vi "Main FPGA.vi"() -> ()   [LabVIEW 2019]
uses:
  Program Files (x86)/National Instruments/LabVIEW 2019/examples/CompactRIO/FPGA Fundamentals/FPGA Math and Analysis/FFT/Type Definitions/Windows.ctl
  <vilib>/Platform/TimedLoop/XDataNode/timing_clust.ctl
  <vilib>/Platform/TimedLoop/XDataNode/nitl_modes.ctl
  <vilib>/Platform/TimedLoop/XDataNode/wakeup.ctl
  <vilib>/rvi/Analysis/measure/FFT/simModelSupport/niFPGA FFT Sim Properties.ctl
  <vilib>/rvi/Analysis/measure/FFT/simModelSupport/niFPGA FFT Sim Types.ctl
  <vilib>/rvi/Analysis/measure/FFT/simModelSupport/niFpgaFFTSimArithmeticProperties.ctl
  <vilib>/rvi/Analysis/measure/FFT/simModelSupport/niFpgaFFTSimDfxp.ctl
  <vilib>/fxp/LVFixedPointQuantizationPolicyTypeDef.ctl
  <vilib>/rvi/Emulation/niFpgaGetClockAttributes.vi
  <vilib>/rvi/Emulation/niFpgaSctlEmulationGetInTimedLoop.vi
  <vilib>/rvi/Emulation/niFpgaEmulationReportErrorSimple.vi
  <vilib>/rvi/Emulation/niFpgaProcessEmulError.vi
  <vilib>/rvi/eio/common/nirviEmuTemplateMethod_errors.vi
  <vilib>/rvi/DataTransferAndStorage/Container/Common/niFpgaContainerExecOnDevCompGetState.vi
  <vilib>/rvi/Emulation/niFpgaEmulationIsFPGAContextNoSignature.vi
  <vilib>/rvi/DataTransferAndStorage/Container/Common/niFpgaContainerGetUniqueNameForEmu.vi
  <vilib>/rvi/errors/nirviReportUnexpectedCaseInternalError (U32).vi
  <vilib>/rvi/Memory/Memory_Emulation/niFpgaMemoryEmulationCacheClearOnFirstRun.vi
  <vilib>/rvi/Memory/Memory_Emulation/nirvimemoryEmulationManagerCache_MakeExclusive.vi
  <vilib>/rvi/Memory/Memory_Emulation/niFpgaMemoryEmulationValidateCache.vi
  <vilib>/rvi/Memory/Memory_Emulation/nirvimemoryEmulationManagerCache_InsertValue.vi
  <vilib>/Utility/error.llb/Clear Errors.vi
  <vilib>/rvi/Memory/Memory_Emulation/nirvimemoryEmulationManagerCache_ReleaseExclusive.vi
  <vilib>/rvi/Memory/Memory_Emulation/nirvimemoryEmulationManagerCache_GetValue.vi
  <vilib>/rvi/Memory/Memory_Emulation/nirvimemoryEmulationManagerCache_SetValue.vi
  <vilib>/rvi/Emulation/niFpgaSctlEmulationResourceMgr.vi
  <vilib>/rvi/Emulation/niFpgaCriticalErrorInLSC.vi
  <vilib>/rvi/errors/niFpgaSetErrorForExecOnDevCompSimple.vi
  <vilib>/rvi/eio/common/nirviEmuReportErrorAndStop.vi
  <vilib>/rvi/FIFO/Fifo_Resource/nirvififoEmulationSetSize.vi
  <vilib>/rvi/FIFO/Fifo_Resource/nirviFifoEmulationQueueMgr.vi
  <instcachedir>/0/nirviFifoEmulationQueueMgr_E5CAEC123FF24DC58D834DCA3CDAA9B5.lvgen/nirviFifoEmulationQueueMgr_E5CAEC123FF24DC58D834DCA3CDAA9B5_002.vi
  <vilib>/rvi/FIFO/Fifo_Resource/nirvififoEmulationDetermineInputValidOut.vi
  <vilib>/rvi/FIFO/Fifo_Resource/nirvififoEmulationCreateLock.vi
  <vilib>/rvi/FIFO/Fifo_Resource/nirvififoEmulationObtainLock.vi
  <vilib>/rvi/FIFO/Fifo_Resource/nirvififoEmulationReleaseLock.vi
  <vilib>/rvi/occurrence/nirviWaitOnOccurrenceBase.vi
  <vilib>/rvi/errors/nirviReportUnexpectedCaseInternalError.vi
  <vilib>/rvi/interface/RandomDataEmulation/niFpgaRandomDataHandleErrors.vi
  <vilib>/rvi/DataTransferAndStorage/Container/Common/niFpgaContainerSetEmuInfo.vi
  <instcachedir>/0/nirviFifoEmulationQueueMgr_E5CAEC123FF24DC58D834DCA3CDAA9B5.lvgen/nirviFifoEmulationQueueMgr_E5CAEC123FF24DC58D834DCA3CDAA9B5_003.vi
  <vilib>/rvi/Analysis/measure/FFT/simModelSupport/niFpgaFFTSimModelCore.vi
  <vilib>/eio/EIONode/EIONode.xnode
  <vilib>/rvi/DataTransferAndStorage/Container/XNode/niFpgaContainer.xnode
  <vilib>/rvi/Memory/Memory_Emulation/niFpgaMemoryEmulationRefIn.vi
  <vilib>/rvi/FIFO/Fifo_Resource/niFpgaFifoEmulationRefIn.vi
  <vilib>/rvi/LocalResourceManager/LocalResourceManager.xnode
  <vilib>/Platform/TimedLoop/XDataNode/XDataNode.xnode
  <vilib>/rvi/interface/RandomDataEmulation/nirviRandomDataFpgaReadWriteTemplate.vi
  <vilib>/rvi/Analysis/measure/FFT/XNode/niFpgaFFT.xnode
  <vilib>/Platform/TimedLoop/XDataNode/XDNodeRunTimeDep.lvlib
panel:
  in  "Number Of Elements":i32=192
  in  "Requested Sample Period (ticks)":u32=1000
  out "Invalid Period":bool
  out "Actual Sample Period (ticks)":u32
  out "Overflow":bool
  in  "Window select":T1=enum."None"
  in  "Update":bool
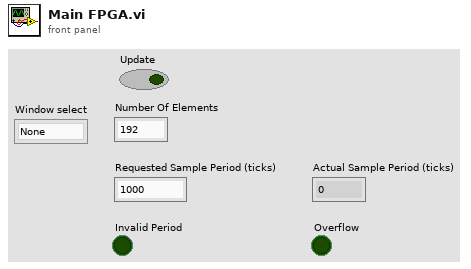
[diagram p1: front panel]
types:
  T1 = typedef "Windows.ctl" = enum16{"Hamming", "Hanning", "None"}
  T2 = typedef "XDNodeRunTimeDep.lvlib/timing_clust.ctl" = cluster{"Expected End [f-1]":u64, "Actual End [f-1]":u64, "Finished Late? [f-1]":bool, "Expected End [i-1]":u64, "Actual End [i-1]":u64, "Finished Late? [i-1]":bool, "Expected Start [i]":u64, "Actual Start [i]":u64, "Expected Start [f]":u64, "Actual Start [f]":u64, "Source Name":string, "Structure Name":string, "Period":i64, "Deadline":i64, "Offset":i64, "Start":i64, "Priority":i32, "Timeout":i32, "Mode":T3, "Wakeup Reason":T4, "Error":errorcluster, "Source Type":string, "Secondary Source Type":string, "Global End Time":u64, "Global Start Time":u64, "Frame Duration":u64, "Iteration Duration":u64, "Assigned CPU":i32, "I/O Scan Engine Mode":u32}
  T3 = typedef "XDNodeRunTimeDep.lvlib/nitl_modes.ctl" = enum32{"No Change", "Process missed periods, maintain original phase", "Discard missed periods, maintain original phase", "Process missed periods, ignore original phase", "Discard missed periods, ignore original phase"}
  T4 = typedef "XDNodeRunTimeDep.lvlib/wakeup.ctl" = enum32{"Normal", "Aborted", "Asynchronous wakeup", "Timing source error", "Timed loop error", "Timeout"}
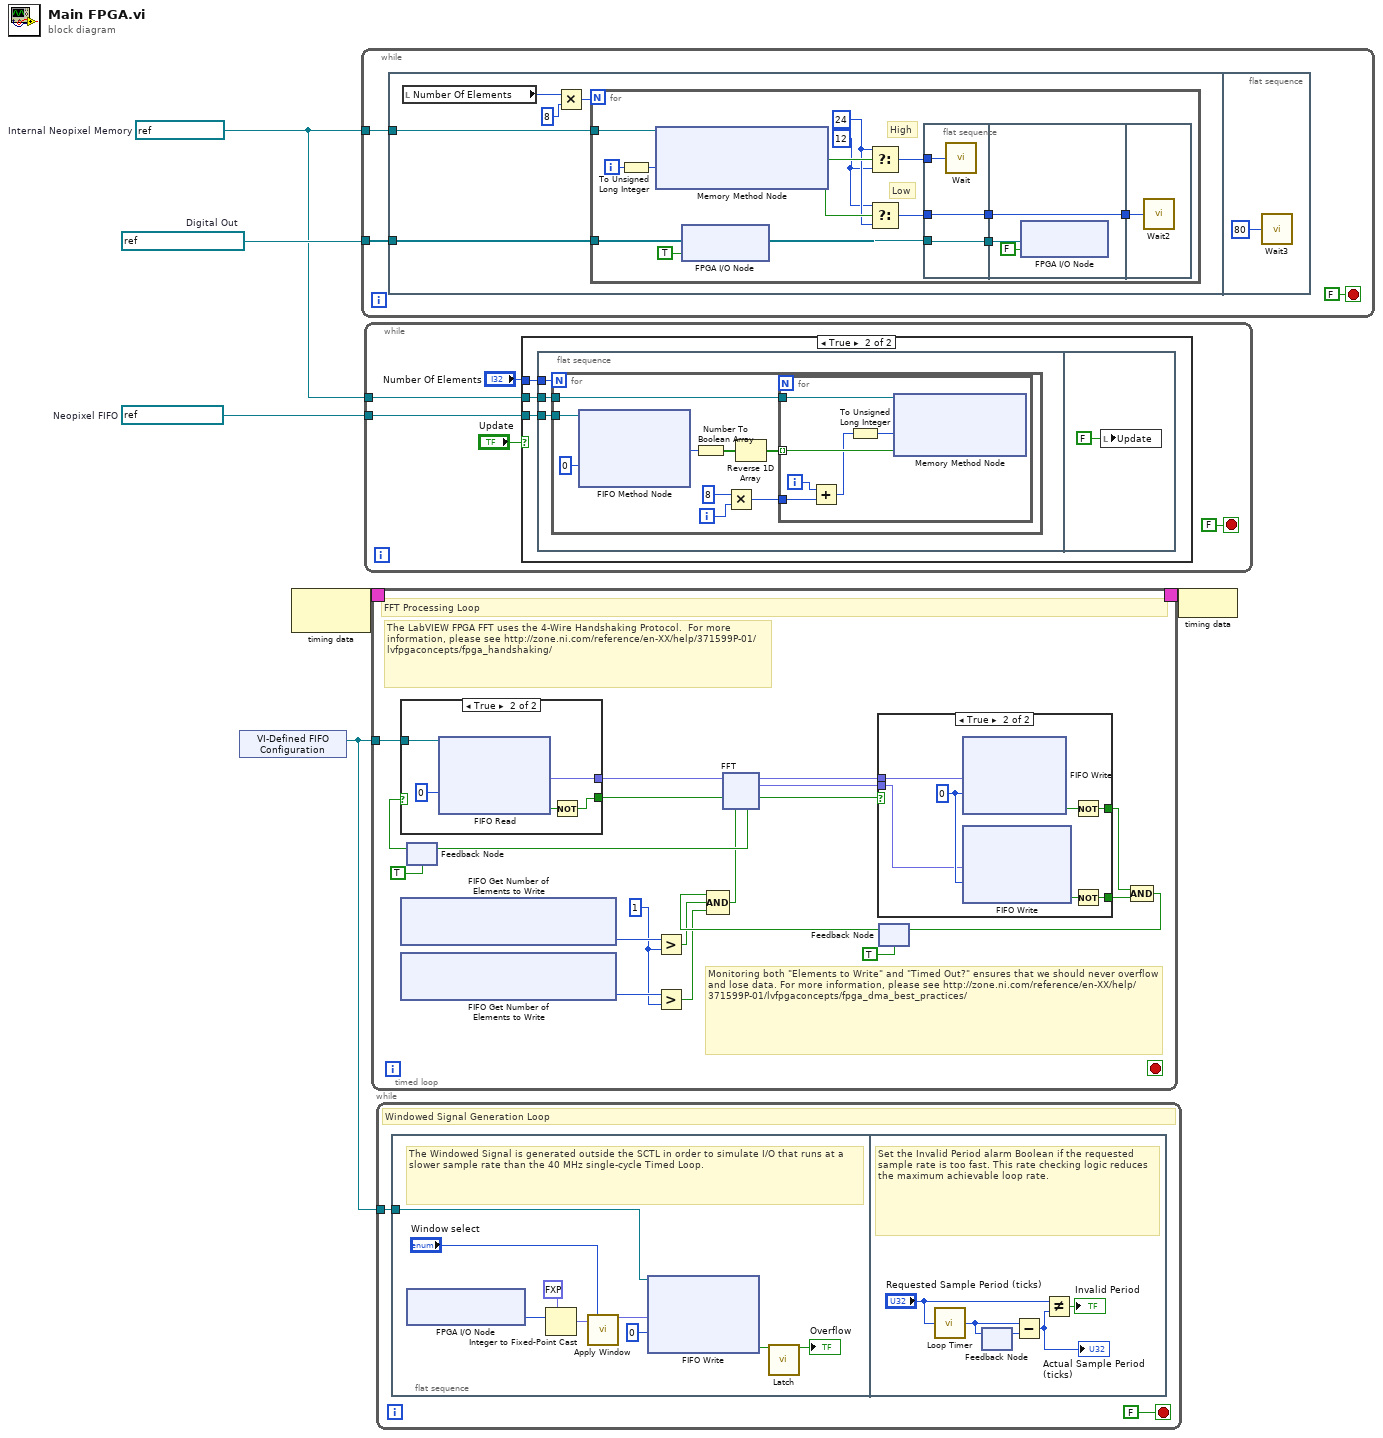
[diagram p0: block diagram]
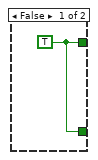
[diagram p2: hidden frame]
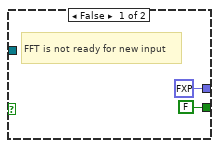
[diagram p3: hidden frame]
diagram:
  w2 = refnum<k21> "Matrix Data"  # Internal Neopixel Memory
  w3 = refnum<k21> "Neopixel FIFO"  # Neopixel FIFO
  w4 = refnum<k21> "ConnectorC/DIO0"  # Digital Out
  n1 = xnode "VI-Defined FIFO Configuration"() -> ("FIFO Out"=w1:refnum<k21>)
  n2 = node-c288() -> (w6:T2)  [unwired: 1 in]
  n3 = while {
    tunnel: w4 -> [w8]
    tunnel: w2 -> [w7]
    stop <- FALSE stop-if-true
    n4 = flat-sequence {
      tunnel: w8 -> [w14]
      tunnel: w7 -> [w11]
      frame #0 {
        n5 = local read "Number Of Elements"() -> (w10:i32)
        n6 = Multiply(x=w10, y=8) -> (x*y=w12:i32)
        n7 = for {
          N: w12 -> [_]
          tunnel: w14 -> [w19]
          tunnel: w11 -> [w15]
          i -> [w27]
          w16 = u8 12 ("High False")
          w17 = u8 24 ("High True")
          # "Low"
          # "High"
          n8 = To Unsigned Long Integer(number=w27) -> (unsigned 32bit integer=w28:u32)
          n9 = xnode ("Memory Method Node")("Address"=w28, "Memory In"=w15) -> ("Data"=w24:bool)  [unwired: 1 out]
          n10 = xnode "FPGA I/O Node"("I/O Item"=TRUE, "FPGA I/O In"=w19) -> ("FPGA I/O Out"=w18:refnum<k21>)
          n11 = Select(t=w17, s=w24, f=w16) -> (s? t:f=w25:u8)
          n12 = Select(t=w16, s=w24, f=w17) -> (s? t:f=w23:u8)
          n13 = flat-sequence {
            tunnel: [w30] -> w26
            tunnel: [w31] -> w21
            tunnel: w23 -> [w31]
            tunnel: w25 -> [w29]
            tunnel: w18 -> [w30]
            tunnel: w26 -> [w34]
            tunnel: [w32] -> w22
            tunnel: w21 -> [w32]
            tunnel: w22 -> [w35]
            frame #0 {
              n14 = call "Wait"("Count(Ticks)"=w29) -> ()  [unwired: 1 out]
            }
            frame #1 {
              n15 = xnode "FPGA I/O Node"("I/O Item"=FALSE, "FPGA I/O In"=w34) -> ()  [unwired: 1 out]
            }
            frame #2 {
              n16 = call "Wait2"("Count(Ticks)"=w35) -> ()  [unwired: 1 out]
            }
          }
        }
      }
      frame #1 {
        n17 = call "Wait3"("Count(uSec)"=u16 80 ("Reset (us)")) -> ()  [unwired: 1 out]
      }
    }
  }
  n18 = while {
    tunnel: w3 -> [w39]
    tunnel: w2 -> [w38]
    stop <- FALSE stop-if-true
    n19 = case shown="True" "Update" {
      tunnel: w39 -> [_ w44]
      tunnel: w38 -> [_ w43]
      tunnel: "Number Of Elements" -> [_ w42]
      frame False {
      }
      frame True {
        n20 = flat-sequence {
          tunnel: w44 -> [w47]
          tunnel: w43 -> [w46]
          tunnel: w42 -> [w45]
          frame #0 {
            n21 = for {
              N: w45 -> [_]
              tunnel: w47 -> [w50]
              tunnel: w46 -> [w48]
              i -> [w56]
              n22 = xnode ("FIFO Method Node")("Timeout"=0, "FIFO In"=w50) -> ("Element"=w51:u8)  [unwired: 2 out]
              n23 = Number To Boolean Array(number=w51) -> (Boolean array=w53:bool[])
              n24 = Multiply(x=8, y=w56) -> (x*y=w54:i32)
              n25 = Reverse 1D Array(array=w53) -> (reversed array=w52:bool[])
              n26 = for {
                tunnel: w52 -> [w61] mode=indexing
                tunnel: w54 -> [w59]
                tunnel: w48 -> [w57]
                i -> [w60]
                n27 = Add(x=w60, y=w59) -> (x+y=w58:i32)
                n28 = To Unsigned Long Integer(number=w58) -> (unsigned 32bit integer=w62:u32)
                n29 = xnode ("Memory Method Node")("Address"=w62, "Data"=w61, "Memory In"=w57) -> ()  [unwired: 1 out]
              }
            }
          }
          frame #1 {
            n30 = local write "Update"(FALSE ("Update")) -> ()
          }
        }
      }
    }
  }
  n31 = timed-loop {
    timing: w6 -> [_]
    timing-out: [_] -> w5
    tunnel: w1 -> [w79]
    stop <- _ stop-if-true
    w69 = u32 1 ("y")
    # "Monitoring both \"Elements to Write\" and \"Timed Out?\" ensures that we should never overflow and lose data. For more information, please see http://zone.ni.com/reference/en-XX/help/371599P-01/lvfpgaconcepts/fpga_dma_best_practices/"
    # "The LabVIEW FPGA FFT uses the 4-Wire Handshaking Protocol.  For more information, please see http://zone.ni.com/reference/en-XX/help/371599P-01/lvfpgaconcepts/fpga_handshaking/"
    # "FFT Processing Loop"
    n32 = xnode ("FIFO Get Number of Elements to Write")() -> ("Number of Elements to Write"=w71:u32)  [unwired: 1 in, 1 out]
    n33 = xnode ("FIFO Get Number of Elements to Write")() -> ("Number of Elements to Write"=w70:u32)  [unwired: 1 in, 1 out]
    n34 = feedback #1(TRUE ("ready for input")) -> (w83:bool)
    n35 = case shown="True" w83 {
      tunnel: [FALSE w123] -> w80
      tunnel: [fxp<+/-,16,5> 0.0 ("Element") w124] -> w82
      tunnel: w79 -> [_ w120]
      frame False {
        # "FFT is not ready for new input"
      }
      frame True {
        n36 = xnode ("FIFO Read")("Timeout"=0, "FIFO In"=w120) -> ("Element"=w124:fxp<+/-,16,5>, "Timed Out?"=w122:bool)  [unwired: 1 out]
        n37 = Not(x=w122) -> (.not. x?=w123:bool)
      }
    }
    n38 = Greater?(x=w71, y=w69) -> (0:w66:bool)
    n39 = Greater?(x=w70, y=w69) -> (0:w65:bool)
    n40 = feedback #2(TRUE) -> (w67:bool)
    n41 = Compound Arithmetic op=AND(w67, w66, w65) -> (w68:bool)
    n42 = xnode "FFT"("real data in"=w82, "input valid"=w80, "ready for output"=w68) -> ("ready for input"=w81:bool, "real data out"=w78:fxp<+/-,25,14>, "imaginary data out"=w77:fxp<+/-,25,14>, "output valid"=w76:bool)  [unwired: 2 in, 1 out]
    n43 = feedback-in #1(w81) -> ()
    n44 = case shown="True" w76 {
      tunnel: w78 -> [_ w112]
      tunnel: w77 -> [_ w111]
      tunnel: [w110 w114] -> w75
      tunnel: [w110 w113] -> w74
      frame False {
        w110 = TRUE ("Timed Out?")
      }
      frame True {
        w117 = 0 ("Timeout")
        n45 = xnode ("FIFO Write")("Element"=w112, "Timeout"=w117) -> ("Timed Out?"=w116:bool)  [unwired: 1 in, 1 out]
        n46 = xnode ("FIFO Write")("Element"=w111, "Timeout"=w117) -> ("Timed Out?"=w115:bool)  [unwired: 1 in, 1 out]
        n47 = Not(x=w116) -> (.not. x?=w114:bool)
        n48 = Not(x=w115) -> (.not. x?=w113:bool)
      }
    }
    n49 = Compound Arithmetic op=AND(w75, w74) -> (w73:bool)
    n50 = feedback-in #2(w73) -> ()
  }
  n51 = while {
    tunnel: w1 -> [w128]
    stop <- FALSE stop-if-true
    # "Windowed Signal Generation Loop"
    n52 = flat-sequence {
      tunnel: w128 -> [w134]
      frame #0 {
        # "The Windowed Signal is generated outside the SCTL in order to simulate I/O that runs at a slower sample rate than the 40 MHz single-cycle Timed Loop."
        n53 = xnode "FPGA I/O Node"() -> ("AudioIn/Right"=w131:i16)  [unwired: 1 in, 1 out]
        n54 = Integer to Fixed-Point Cast(fixed-point type=fxp<+/-,16,5> 0.0 ("Signal In"), integer=w131) -> (fixed-point=w129:fxp<+/-,16,5>)
        n55 = call "Apply Window.vi"("Signal In"=w129, "Window select"="Window select") -> ("Windowed Signal Out"=w135:fxp<+/-,16,5>)  [unwired: 13 in]
        n56 = xnode ("FIFO Write")("Element"=w135, "Timeout"=0, "FIFO In"=w134) -> ("Timed Out?"=w133:bool)  [unwired: 1 out]
        n57 = call "Latch.vi"("Input"=w133) -> ("Output"=→"Overflow":bool)  [unwired: 14 in]
      }
      frame #1 {
        # "Set the Invalid Period alarm Boolean if the requested sample rate is too fast. This rate checking logic reduces the maximum achievable loop rate."
        n58 = call "Loop Timer"("Count(Ticks)"="Requested Sample Period (ticks)") -> ("Tick Count(Ticks)"=w138:u32)
        n59 = feedback #3() -> (w139:u32)  [unwired: 1 in]
        n60 = feedback-in #3(w138) -> ()
        n61 = Subtract(x=w138, y=w139) -> (x-y=w142:u32)
        "Actual Sample Period (ticks)" <- w142
        n62 = Not Equal?(x="Requested Sample Period (ticks)", y=w142) -> (x != y?=→"Invalid Period":bool)
      }
    }
  }
  n63 = node-c288(w5) -> ()
